vi "LESSON2_PROJECT1.vi"() -> ()   [LabVIEW 2022 SP3]
panel:
  out "C":dbl
  in  "B":dbl
  in  "A":dbl
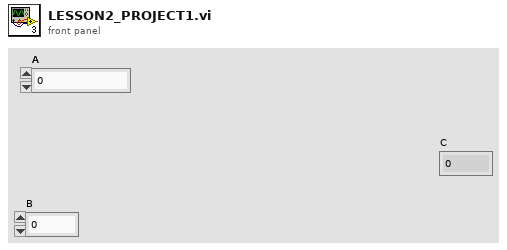
[diagram p1: front panel]
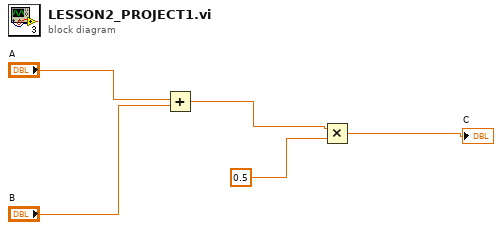
[diagram p0: block diagram]
diagram:
  n1 = Add(x="A", y="B") -> (x+y=w3:dbl)
  n2 = Multiply(x=w3, y=0.5) -> (x*y=→"C":dbl)
